vi "WPI_ADI_IMU_AHRS_RoboBees.vi"(8 "Yaw Axis":enum16{"X", "Y", "Z"}(ring)=enum."Z", 9 "dt (s)":dbl, 10 "IMU Rates":T1) -> (0 "Yaw":dbl(knob) scale=-180.0..180.0, 1 "Roll":dbl(knob) scale=-180.0..180.0, 2 "Pitch":dbl(knob) scale=-90.0..90.0, 3 "Output":dbl[](array[numeric]))   [LabVIEW 2015, in "FRC ADI MXP IMU.lvlib"]
uses:
  FRC ADI MXP IMU.lvlib
panel:
  in  "Tilt Comp (Yaw)":bool
  in  "tau mag":dbl=0.04
  in  "tau acc":dbl=0.6
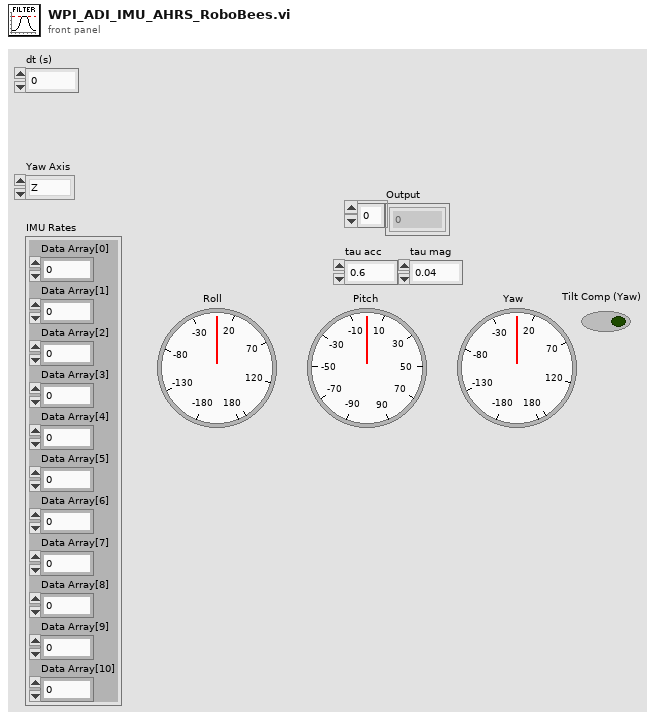
[diagram p1: front panel]
types:
  T1 = cluster{"Data Array[0]":dbl, "Data Array[1]":dbl, "Data Array[2]":dbl, "Data Array[3]":dbl, "Data Array[4]":dbl, "Data Array[5]":dbl, "Data Array[6]":dbl, "Data Array[7]":dbl, "Data Array[8]":dbl, "Data Array[9]":dbl, "Data Array[10]":dbl}
  T2 = cluster{"Xaccel":dbl, "Yaccel":dbl, "Zaccel":dbl}
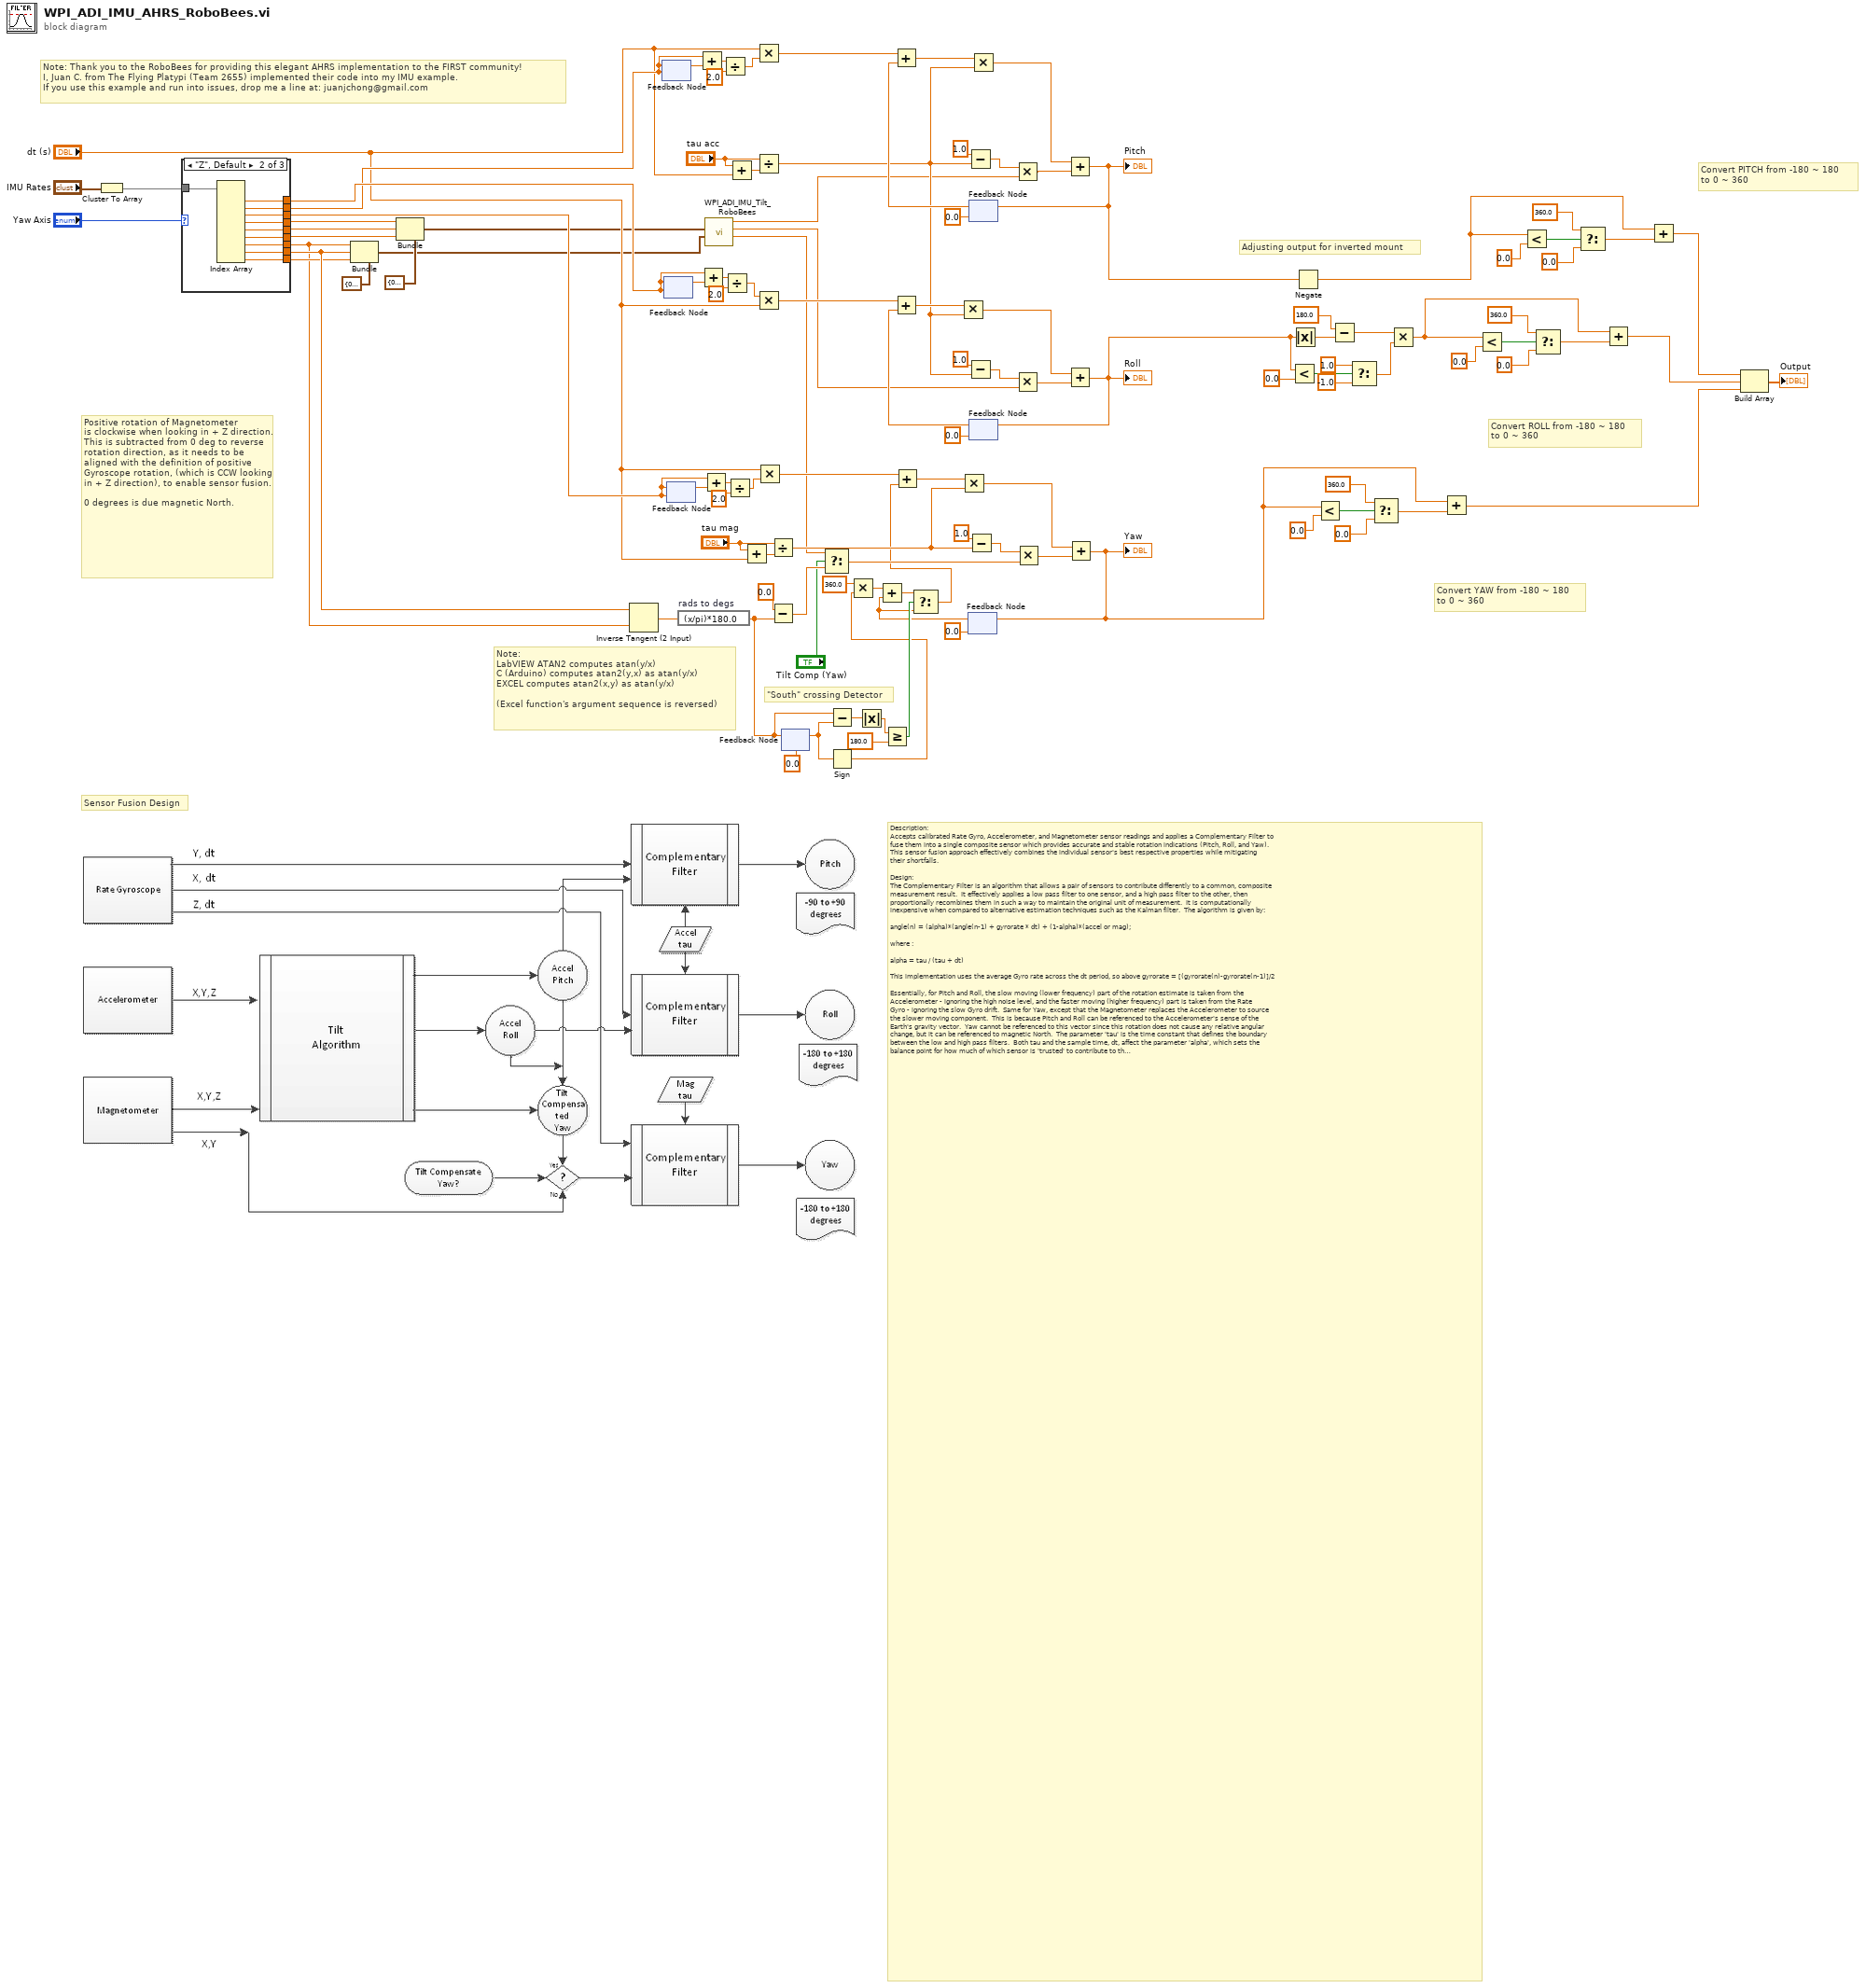
[diagram p0: block diagram]
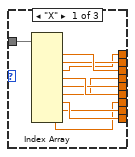
[diagram p2: hidden frame]
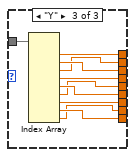
[diagram p3: hidden frame]
diagram:
  # "Convert PITCH from -180 ~ 180 \nto 0 ~ 360"
  # "Convert ROLL from -180 ~ 180 \nto 0 ~ 360"
  # "Convert YAW from -180 ~ 180 \nto 0 ~ 360"
  # "Note: Thank you to the RoboBees for providing this elegant AHRS implementation to the FIRST community!\nI, Juan C. from The Flying Platypi (Team 2655) implemented their code into my IMU example.\nIf you use this example and run into issues, drop me a line at: juanjchong@gmail.com"
  # "Adjusting output for inverted mount"
  # "Sensor Fusion Design"
  # "Description:\nAccepts calibrated Rate Gyro, Accelerometer, and Magnetometer sensor readings and applies a Complementary Filter to\nfuse them into a single composite sensor which provides accurate and stable rotation indications (Pitch, Roll, and Yaw).\nThis sensor fusion approach effectively combines the individual sensor's best respective properties while mitigating\ntheir shortfalls.\n\nDesign:\nThe Complementary Filter is an algorithm that allows a pair of sensors to contribute differently to a common, composite\nmeasurement result.  It effectively applies a low pass filter to one sensor, and a high pass filter to the other, then\nproportionally recombines them in such a way to maintain the original unit of measurement.  It is computationally\ninexpensive when compared to alternative estimation techniques such as the Kalman filter.  The algorithm is given by:\n\nangle(n) = (alpha)*(angle(n-1) + gyrorate * dt) + (1-alpha)*(accel or mag);\n\nwhere : \n\nalpha = tau / (tau + dt)\n\nThis implementation uses the average Gyro rate across the dt period, so above gyrorate = [(gyrorate(n)-gyrorate(n-1)]/2\n\nEssentially, for Pitch and Roll, the slow moving (lower frequency) part of the rotation estimate is taken from the\nAccelerometer - ignoring the high noise level, and the faster moving (higher frequency) part is taken from the Rate \nGyro - ignoring the slow Gyro drift.  Same for Yaw, except that the Magnetometer replaces the Accelerometer to source\nthe slower moving component.  This is because Pitch and Roll can be referenced to the Accelerometer's sense of the\nEarth's gravity vector.  Yaw cannot be referenced to this vector since this rotation does not cause any relative angular\nchange, but it can be referenced to magnetic North.  The parameter 'tau' is the time constant that defines the boundary\nbetween the low and high pass filters.  Both tau and the sample time, dt, affect the parameter 'alpha', which sets the\nbalance point for how much of which sensor is 'trusted' to contribute to the rotation estimate.\n\nThe Complementary Filter algorithm is applied to each X/Y/Z rotation axis to compute R/P/Y outputs, respectively.\n\nMagnetometer readings are tilt-compensated when Tilt-Comp-(Yaw) is asserted (True), by the IMU TILT subVI.  This\ncreates what is known as a tilt-compensated compass, which allows Yaw to be insensitive to the effects of a\nnon-level sensor, but generates error in Yaw during movement (coordinate acceleration).\n\nThe Yaw \"South\" crossing detector is necessary to allow a smooth transition across the +/- 180 deg discontinuity (inherent\nin the ATAN function).  Since -180 deg is congruent with +180 deg, Yaw needs to jump between these values when\ncrossing South (North is 0 deg).  The design depends upon comparison of successive Yaw readings to detect a cross-over\nevent.  The cross-over detector monitors the current reading and evaluates how far it is from the previous reading.  If it\nis greater than the previous reading by the Discriminant (= 180 deg), then Yaw just crossed South.\n\nBy choosing 180 as the Discriminant, the only way the detector can produce a false positive, assuming a loop iteration\nof 70 msec, is for it to rotate >2,571 dps ... (2,571=180/.07).  This is faster than the ST L3GD20 Gyro can register.  The\ndetector produces a Boolean True upon detecting a South crossing.  This is used to alter the (n-1) Yaw which was\npreviously stored, either adding or subtracting 360 degrees as required to place the previous Yaw in the correct quadrant\nwhenever crossing occurs.  The Modulus function cannot be used here as the Complementary Filter algorithm has 'state'\n(needs to remember previous Yaw).\n \nWe are in effect stitching together two ends of a ruler for 'modular arithmetic' (clock math).\n\nInputs:\nGYRO - Gyro rate and sample time measurements.\nACCEL - Acceleration measurements.\nMAG - Magnetic measurements.\nTAU ACC - tau parameter used to set sensor balance between Accel and Gyro for Roll and Pitch.\nTAU MAG -  tau parameter used to set sensor balance between Mag and Gyro for Yaw.\nTILT COMP (Yaw) - Enables Yaw tilt-compensation if True.\n\nOutputs:\nROLL - Filtered Roll about sensor X-axis.\nPITCH - Filtered Pitch about sensor Y-axis.\nYAW - Filtered Yaw about sensor Z-axis.\n\nVI Properties:\nExecution Reentrancy is set to Non Reentrant Execution\n\nImplementation:\nIt's best to establish the optimum loop sample time first.  See IMU READ implementation notes for guidance.  Each\ntau parameter should then be adjusted to achieve optimum sensor fusion.  tau acc affects Roll and Pitch, tau mag affects\nYaw.  Start at value 1 or 2 and decrease by half each time until the result doesn't drift, but not so far that the result gets\nnoisy.  An optimum tau for this IMU is likely in the range of 1.0 to 0.01, for a loop sample time between 10 and 100 ms.\n\nNote that both sample timing (dt) and tau both affect the balance parameter, 'alpha'.  Adjusting either dt or tau will\nrequire the other to be readjusted to maintain a particular filter performance.\n\nIt is likely best to set Yaw tilt-compensation to off (False) if the Yaw value is to be used as feedback in a closed loop\ncontrol application.  The tradeoff is that Yaw will only be accurate while the robot is level.\n\nSince a Yaw of -180 degrees is congruent with +180 degrees (they represent the same direction), it is possible that the\nYaw output will oscillate between these two values when the sensor happens to be pointing due South, as sensor\nnoise causes slight variation.  You will need to account for this possibility if you are using the Yaw value for decision-\nmaking in code.\n\n----- The RoboBees FRC Team 836! -----  Complement your passion to solve problems with a STEM Education!"
  # "\"South\" crossing Detector"
  # "Positive rotation of Magnetometer\nis clockwise when looking in + Z direction.  This is subtracted from 0 deg to reverse rotation direction, as it needs to be aligned with the definition of positive Gyroscope rotation, (which is CCW looking in + Z direction), to enable sensor fusion.\n\n0 degrees is due magnetic North."
  # "Note:\nLabVIEW ATAN2 computes atan(y/x)\nC (Arduino) computes atan2(y,x) as atan(y/x)\nEXCEL computes atan2(x,y) as atan(y/x)\n\n(Excel function's argument sequence is reversed)"
  n1 = Cluster To Array(cluster="IMU Rates") -> (array=w50:dbl[])
  n2 = case shown="\"Z\", Default" "Yaw Axis" {
    tunnel: [w118 w131 w140] -> w49
    tunnel: [w115 w130 w137] -> w41
    tunnel: w50 -> [w121 w129 w141]
    tunnel: [w112 w128 w134] -> w43
    tunnel: [w116 w127 w135] -> w40
    tunnel: [w117 w126 w136] -> w39
    tunnel: [w119 w125 w138] -> w48
    tunnel: [w120 w124 w139] -> w47
    tunnel: [w113 w123 w132] -> w45
    tunnel: [w114 w122 w133] -> w44
    frame "X" {
      n3 = Index Array(array=w121) -> (element #1=w120:dbl, element #2=w119:dbl, element #3=w118:dbl, element #4=w117:dbl, element #5=w116:dbl, element #6=w115:dbl, element #7=w114:dbl, element #8=w113:dbl, element #9=w112:dbl)  [unwired: 9 in]
    }
    frame "Z", Default {
      n4 = Index Array(array=w129) -> (element #1=w131:dbl, element #2=w125:dbl, element #3=w124:dbl, element #4=w130:dbl, element #5=w127:dbl, element #6=w126:dbl, element #7=w128:dbl, element #8=w123:dbl, element #9=w122:dbl)  [unwired: 9 in]
    }
    frame "Y" {
      n5 = Index Array(array=w141) -> (element #1=w140:dbl, element #2=w139:dbl, element #3=w138:dbl, element #4=w137:dbl, element #5=w136:dbl, element #6=w135:dbl, element #7=w134:dbl, element #8=w133:dbl, element #9=w132:dbl)  [unwired: 9 in]
    }
  }
  n6 = Bundle(cluster=cluster{"Xmag":dbl, "Ymag":dbl, "Zmag":dbl} {"Xmag"=0.0, "Ymag"=0.0, "Zmag"=0.0} ("Mag"), "Xmag"=w43, "Ymag"=w45, "Zmag"=w44) -> (w36:cluster{"Xmag":dbl, "Ymag":dbl, "Zmag":dbl})
  n7 = Bundle(cluster=T2 {"Xaccel"=0.0, "Yaccel"=0.0, "Zaccel"=0.0} ("Accel"), "Xaccel"=w41, "Yaccel"=w40, "Zaccel"=w39) -> (w37:T2)
  n8 = Inverse Tangent (2 Input)(1:w43, 2:w45) -> (0:w84:dbl)
  n9 = feedback #1(w48) -> (w73:dbl)
  n10 = feedback-in #1(w48) -> ()
  n11 = feedback #2(w49) -> (w67:dbl)
  n12 = feedback-in #2(w49) -> ()
  n13 = feedback #3(w47) -> (w65:dbl)
  n14 = feedback-in #3(w47) -> ()
  n15 = expression code="(x/pi)*180.0" "rads to degs"(w84) -> (w54:dbl)
  n16 = Add(x=w48, y=w73) -> (x+y=w72:dbl)
  n17 = Add(x=w49, y=w67) -> (x+y=w68:dbl)
  n18 = Add(x=w47, y=w65) -> (x+y=w64:dbl)
  n19 = call "WPI_ADI_IMU_Tilt_RoboBees.vi"("Mag"=w36, "Accel"=w37) -> ("Yaw"=w33:dbl, "Roll"=w34:dbl, "Pitch"=w35:dbl)  [unwired: 6 in, 1 out]
  n20 = Divide(x=w72, y=2.0) -> (x/y=w70:dbl)
  n21 = Divide(x=w68, y=2.0) -> (x/y=w66:dbl)
  n22 = Divide(x=w64, y=2.0) -> (x/y=w62:dbl)
  n23 = Add(x="tau acc", y="dt (s)") -> (x+y=w110:dbl)
  n24 = Add(x="tau mag", y="dt (s)") -> (x+y=w85:dbl)
  n25 = Multiply(x="dt (s)", y=w70) -> (x*y=w98:dbl)
  n26 = Divide(x="tau acc", y=w110) -> (x/y=w94:dbl)
  n27 = Multiply(x=w66, y="dt (s)") -> (x*y=w108:dbl)
  n28 = Multiply(x="dt (s)", y=w62) -> (x*y=w78:dbl)
  n29 = Divide(x="tau mag", y=w85) -> (x/y=w77:dbl)
  n30 = Subtract(x=0.0 ("y"), y=w54) -> (x-y=w81:dbl)
  n31 = feedback #4(0.0) -> (w55:dbl)
  n32 = feedback-in #4(w54) -> ()
  n33 = Select(t=w33, s="Tilt Comp (Yaw)", f=w81) -> (s? t:f=w82:dbl)
  n34 = Subtract(x=w54, y=w55) -> (x-y=w61:dbl)
  n35 = Sign(1:w55) -> (0:w57:dbl)
  n36 = Multiply(x=360.0 ("y"), y=w57) -> (x*y=w53:dbl)
  n37 = Absolute Value(x=w61) -> (abs(x)=w60:dbl)
  n38 = Greater Or Equal?(x=w60, y=180.0) -> (x >= y?=w58:bool)
  n39 = Subtract(x=1.0, y=w94) -> (x-y=w97:dbl)
  n40 = Subtract(x=1.0, y=w94) -> (x-y=w93:dbl)
  n41 = Subtract(x=1.0, y=w77) -> (x-y=w91:dbl)
  n42 = feedback #5(0.0) -> (w52:dbl)
  n43 = Add(x=w53, y=w52) -> (x+y=w74:dbl)
  n44 = Select(t=w74, s=w58, f=w52) -> (s? t:f=w75:dbl)
  n45 = Add(x=w78, y=w75) -> (x+y=w88:dbl)
  n46 = Multiply(x=w88, y=w77) -> (x*y=w90:dbl)
  n47 = feedback #6(0.0) -> (w102:dbl)
  n48 = Add(x=w98, y=w102) -> (x+y=w99:dbl)
  n49 = Multiply(x=w99, y=w94) -> (x*y=w101:dbl)
  n50 = feedback #7(0.0) -> (w92:dbl)
  n51 = Add(x=w108, y=w92) -> (x+y=w107:dbl)
  n52 = Multiply(x=w107, y=w94) -> (x*y=w105:dbl)
  n53 = Multiply(x=w97, y=w35) -> (x*y=w100:dbl)
  n54 = Multiply(x=w93, y=w34) -> (x*y=w106:dbl)
  n55 = Multiply(x=w91, y=w82) -> (x*y=w89:dbl)
  n56 = Add(x=w101, y=w100) -> (x+y=w23:dbl)
  "Pitch" <- w23
  n57 = feedback-in #6(w23) -> ()
  n58 = Add(x=w105, y=w106) -> (x+y=w22:dbl)
  "Roll" <- w22
  n59 = feedback-in #7(w22) -> ()
  n60 = Add(x=w90, y=w89) -> (x+y=w16:dbl)
  "Yaw" <- w16
  n61 = feedback-in #5(w16) -> ()
  n62 = Less?(x=w22, y=0.0) -> (x < y?=w28:bool)
  n63 = Absolute Value(x=w22) -> (abs(x)=w31:dbl)
  n64 = Negate(x=w23) -> (-x=w1:dbl)
  n65 = Less?(x=w16, y=0.0) -> (x < y?=w20:bool)
  n66 = Subtract(x=180.0 ("y"), y=w31) -> (x-y=w25:dbl)
  n67 = Select(t=1.0, s=w28, f=-1.0) -> (s? t:f=w24:dbl)
  n68 = Select(t=360.0, s=w20, f=0.0) -> (s? t:f=w17:dbl)
  n69 = Multiply(x=w25, y=w24) -> (x*y=w9:dbl)
  n70 = Add(x=w16, y=w17) -> (x+y=w15:dbl)
  n71 = Less?(x=w9, y=0.0) -> (x < y?=w13:bool)
  n72 = Less?(x=w1, y=0.0) -> (x < y?=w6:bool)
  n73 = Select(t=360.0, s=w13, f=0.0) -> (s? t:f=w10:dbl)
  n74 = Select(t=360.0, s=w6, f=0.0) -> (s? t:f=w3:dbl)
  n75 = Add(x=w9, y=w10) -> (x+y=w8:dbl)
  n76 = Add(x=w1, y=w3) -> (x+y=w2:dbl)
  n77 = Build Array(w2, w8, w15) -> (→"Output":dbl[])
